vi "Read Encryption Type.vi"(8 "error in (no error)":errorcluster, 11 "User Configuration Manager in":refnum<class "User Configuration Manager.lvclass">) -> (0 "error out":errorcluster, 2 "Encryption Type":refnum<class "iEncryption.lvclass">, 3 "User Configuration Manager out":refnum<class "User Configuration Manager.lvclass">)   [LabVIEW 2019, in "User Configuration Manager.lvlib" / "User Configuration Manager.lvclass"]
uses:
  <vilib>/gpm_packages/@cs/user-manager/Source/User Configuration Manager/User Configuration Manager.lvclass
  <vilib>/gpm_packages/@cs/user-manager/Source/iEncryption/iEncryption.lvclass
  <vilib>/gpm_packages/@cs/user-manager/Source/User Configuration Manager/User Configuration Manager.lvclass/User Configuration Manager.ctl
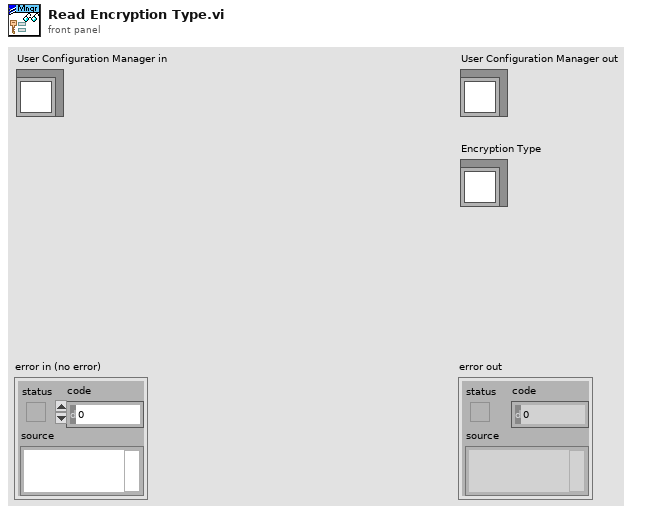
[diagram p1: front panel]
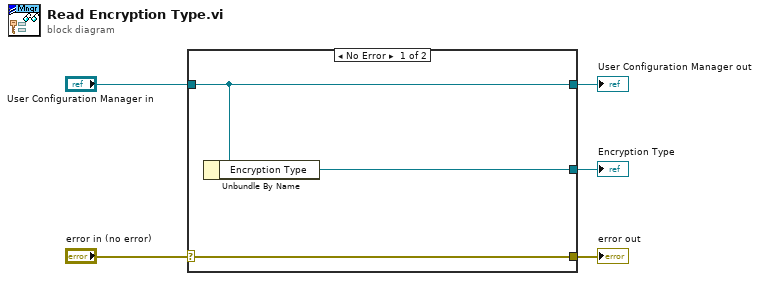
[diagram p0: block diagram]
diagram:
  n1 = case shown="No Error" "error in (no error)" {
    selector: "error in (no error)" -> [w8 w9]
    tunnel: [w8 w9] -> w4
    tunnel: [w7 w10] -> w2
    tunnel: "User Configuration Manager in" -> [w7 w10]
    tunnel: [w6 _] -> w1
    frame No Error {
      n2 = Unbundle By Name(w7) -> ("Encryption Type"=w6:refnum<class "iEncryption.lvclass">)
    }
    frame Error {
    }
  }
  "error out" <- w4
  "User Configuration Manager out" <- w2
  "Encryption Type" <- w1
